vi "Get Class Settings - Get Accessors Scope.vi"(8 "error in (no error)":errorcluster {"code" format="Error %.0f"}, 11 "VIDoc Printer In":refnum<class "VIDoc Printer.lvclass">) -> (0 "error out":errorcluster {"code" format="Error %.0f"}, 2 "Scope Settings":T1={"Public"=TRUE, "Protected"=TRUE, "Community"=TRUE, "Private"=TRUE, "Unknown"=TRUE}, 3 "VIDoc Printer Out":refnum<class "VIDoc Printer.lvclass">)   [LabVIEW 2023, in "VIDoc Printer.lvlib" / "VIDoc Printer.lvclass"]
uses:
  VIDoc Printer.lvclass
  Settings/Printer Settings/Scope Settings.ctl
  Settings/Printer Settings/Printer Settings.lvclass
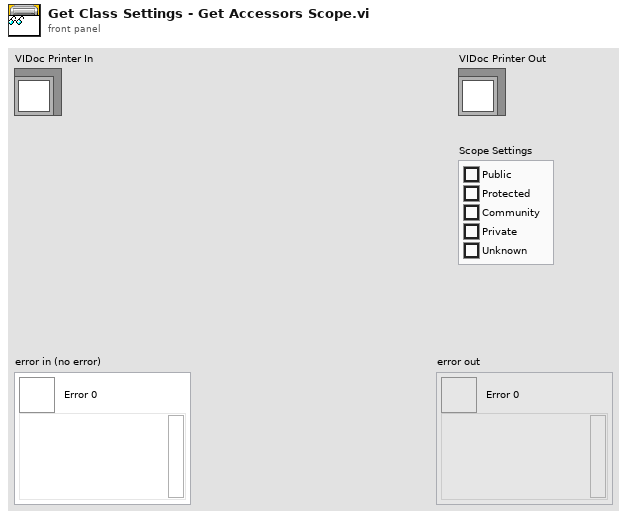
[diagram p1: front panel]
types:
  T1 = typedef "VIDoc Printer.lvlib/Printer Settings.lvclass/Scope Settings.ctl" = cluster{"Public":bool, "Protected":bool, "Community":bool, "Private":bool, "Unknown":bool}
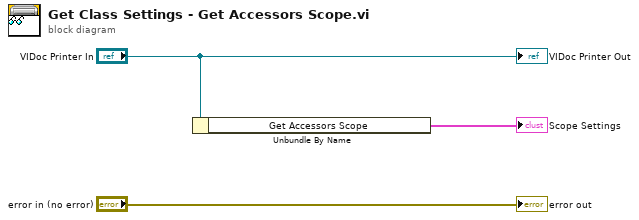
[diagram p0: block diagram]
diagram:
  n1 = Unbundle By Name("VIDoc Printer In") -> ("Get Accessors Scope"=→"Scope Settings":T1)
  "error out" <- "error in (no error)"
  "VIDoc Printer Out" <- "VIDoc Printer In"
